vi "Broadcast Batch Messages.vi"(8 "error in (no error)":errorcluster, 9 "Mail Strategy In":refnum<class "Mail Strategy.lvclass">, 10 "Messages In":refnum<class "Message.lvclass">[](array[class]), 11 "Messenger in":refnum<class "Simple Tree Queue Messenger.lvclass">) -> (0 "error out":errorcluster, 3 "Messenger out":refnum<class "Simple Tree Queue Messenger.lvclass">)   [LabVIEW 2024, in "Simple Tree Queue Messenger.lvclass"]
uses:
  Simple Tree Queue Messenger.lvclass
  Ancestor Class/Message/Message.lvclass
  Ancestor Class/Messenger/Mail Strategy/Mail Strategy.lvclass
  Simple Tree Queue Messenger.lvclass/Simple Tree Queue Messenger.ctl
  Ancestor Class/Messenger/Messenger Composite/Messenger Composite.lvclass/Messenger Composite.ctl
  Ancestor Class/Messenger/Messenger Composite/Public Data/Read Nodes.vi
  Ancestor Class/Messenger/Messenger/Messenger.lvclass
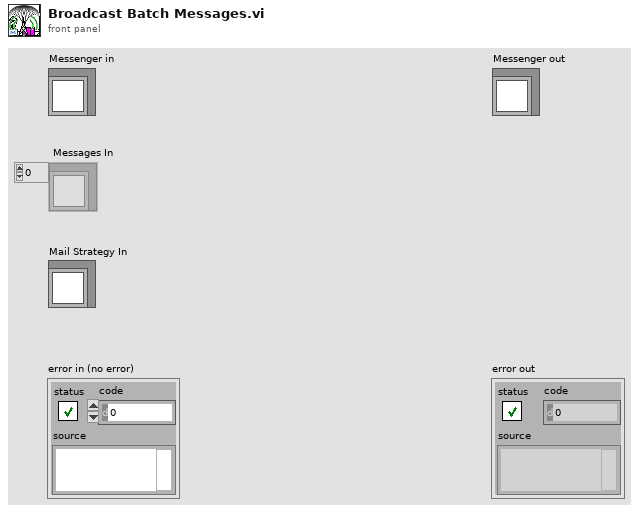
[diagram p1: front panel]
types:
  T1 = typedef "Message Queue.ctl" = refnum<queue>
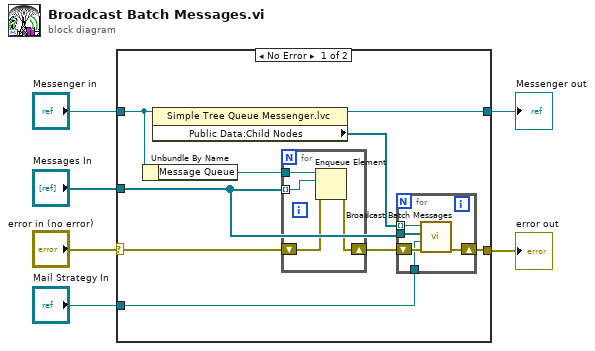
[diagram p0: block diagram]
diagram:
  n1 = case shown="No Error" "error in (no error)" {
    selector: "error in (no error)" -> [w14 w26]
    tunnel: [w12 w26] -> w5
    tunnel: [w8 w25] -> w4
    tunnel: "Messenger in" -> [w10 w25]
    tunnel: "Messages In" -> [w11 _]
    tunnel: "Mail Strategy In" -> [w7 _]
    frame No Error {
      n2 = Unbundle By Name(w10) -> ("Message Queue"=w15:T1)
      n3 = property class="Simple Tree Queue Messenger.lvc"(reference=w10) -> (reference out=w8:refnum<class "Simple Tree Queue Messenger.lvclass">, "Public Data:Child Nodes"=w9:refnum<class "Messenger.lvclass">[])  [unwired: 1 in, 1 out]
      n4 = for {
        tunnel: w15 -> [w24]
        tunnel: w11 -> [w23] mode=indexing
        shift-right: [w21] -> w13
        shift-left: w14 -> [w22]
        n5 = Enqueue Element(queue=w24, element=w23, error in (no error)=w22) -> (error out=w21:errorcluster)  [unwired: 1 in, 2 out]
      }
      n6 = for {
        shift-right: [w17] -> w12
        shift-left: w13 -> [w18]
        tunnel: w9 -> [w20] mode=indexing
        tunnel: w11 -> [w19]
        tunnel: w7 -> [w16]
        n7 = call-dynamic "Broadcast Batch Messages.vi"("error in (no error)"=w18, "Mail Strategy In"=w16, "Messages In"=w19, "Messenger in"=w20) -> ("error out"=w17:errorcluster)  [unwired: 6 in, 1 out]
      }
    }
    frame Error {
    }
  }
  "error out" <- w5
  "Messenger out" <- w4
